vi "BRig_Host_dataRunState_test.vi"() -> ()   [LabVIEW 2014]
panel:
  out "output_updatePlot":bool
  out "output_idx":i32[](array[numeric])
  out "output_dataTS":u16[][](array[numeric])
  out "output_dataPlot":u16[][](array[numeric])
  in  "input_iSelection":u16
  in  "input_tSelectionPlot":u16
  in  "input_tSelection":u16
  in  "input_sSelection":u16
  in  "input_LorR":u16
  in  "input_nTrial":u16
  in  "input_idx":i32[](array[numeric])
  in  "input_dataPlot":u16[][](array[numeric])
  in  "input_dataTS":u16[][](array[numeric])
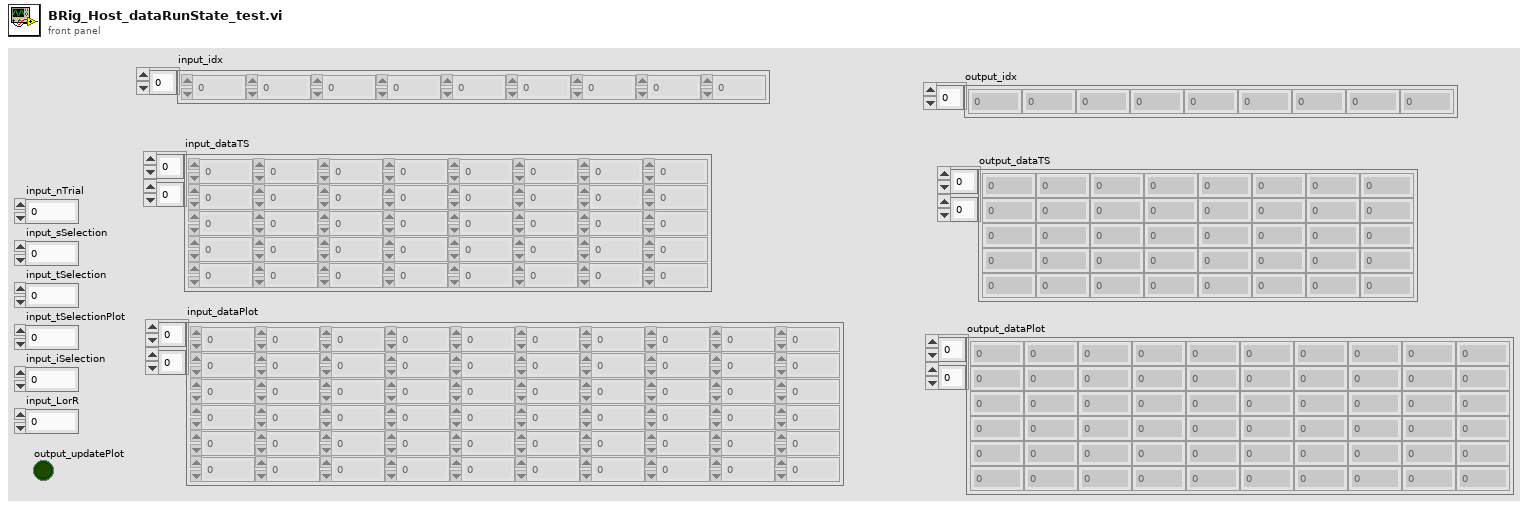
[diagram p1: front panel]
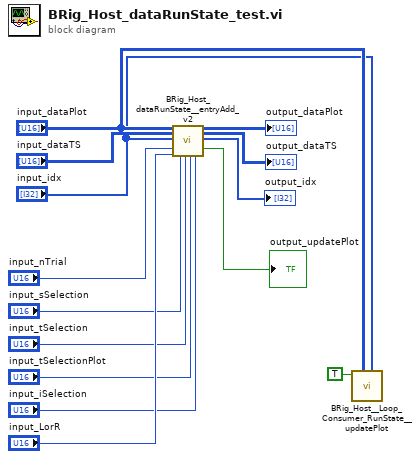
[diagram p0: block diagram]
diagram:
  n1 = call "BRig_Host_dataRunState__entryAdd_v2.vi"("input_dataPlot"="input_dataPlot", "input_dataTS"="input_dataTS", "input_idx"="input_idx", "input_nTrial"="input_nTrial", "input_LorR"="input_LorR", "input_sSelection"="input_sSelection", "input_tSelection"="input_tSelection", "input_tSelectionPlot"="input_tSelectionPlot", "input_iSelection"="input_iSelection") -> ("output_dataPlot"=→"output_dataPlot":u16[][], "output_dataTS"=→"output_dataTS":u16[][], "output_idx"=→"output_idx":i32[], "output_updatePlot"=→"output_updatePlot":bool)  [unwired: 7 in]
  n2 = call "BRig_Host__Loop_Consumer_RunState__updatePlot.vi"("input_idx"="input_idx", "input_dataPlot"="input_dataPlot", "input_updatePlot"=TRUE) -> ()  [unwired: 8 in, 1 out]
